vi "convertToKeyValuePair_integer64bit.vi"(8 "error in (no error)":errorcluster, 10 "value":i64, 11 "name":string) -> (0 "error out":errorcluster, 3 "string converted":string)   [LabVIEW 2018]
doc: "Convert an 64-bit integer numeric into a key value pair as string."
uses:
  convertToKeyValuePair_string.vi
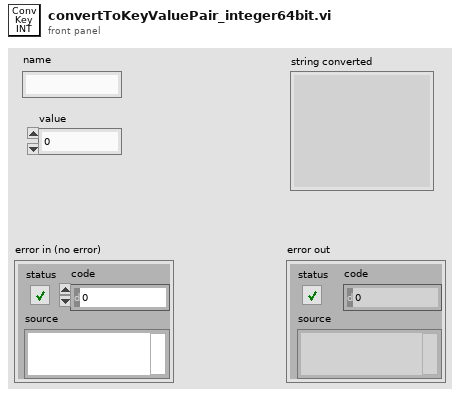
[diagram p1: front panel]
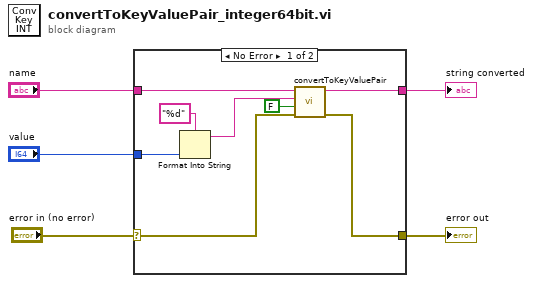
[diagram p0: block diagram]
diagram:
  n1 = case shown="No Error" "error in (no error)" {
    selector: "error in (no error)" -> [w7 w14]
    tunnel: "value" -> [w9 _]
    tunnel: "name" -> [w11 _]
    tunnel: [w6 w14] -> w2
    tunnel: [w10 _] -> w1
    frame No Error {
      n2 = Format Into String(format string="%d", w9) -> (resulting string=w13:string)  [unwired: 2 in, 1 out]
      n3 = call-poly "convertToKeyValuePair.vi"("error in (no error)"=w7, "double quotes (T)"=FALSE, "value"=w13, "name"=w11) -> ("error out"=w6:errorcluster, "string converted"=w10:string)  [unwired: 6 in]
    }
    frame Error {
    }
  }
  "error out" <- w2
  "string converted" <- w1
